vi "Unregister Event.vi"(7 "Event":refnum<class "Event.lvclass">, 8 "error in (no error)":errorcluster, 11 "View in":refnum<class "View.lvclass">) -> (0 "error out":errorcluster, 3 "View out":refnum<class "View.lvclass">)   [LabVIEW 2023, in "MVC Actors.lvlib" / "View.lvclass"]
doc: "Unregisters an event to the Controller by specifiying the concrete event."
uses:
  View.lvclass
  Event/Event.lvclass
  View.lvclass/View.ctl
  properties/Read Controller Actor Enqueuer.vi
  properties/Read Name.vi
  <vilib>/ActorFramework/Message Enqueuer/Message Enqueuer.lvclass
  Controller Messages/Unregister by Name Msg/Unregister by Name Msg.lvclass
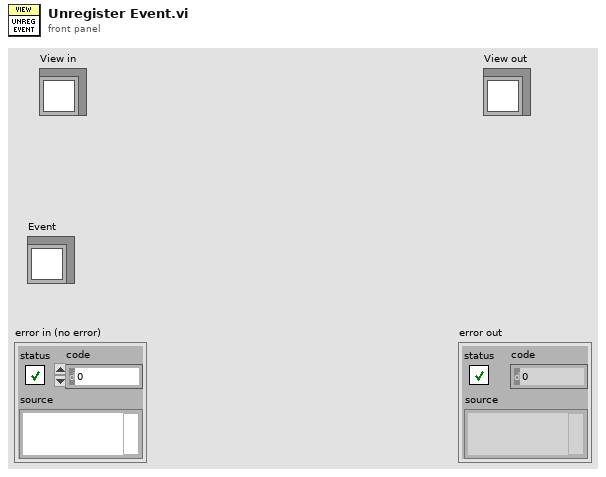
[diagram p1: front panel]
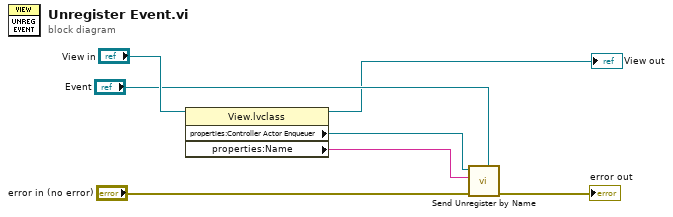
[diagram p0: block diagram]
diagram:
  n1 = property class="View.lvclass"(reference="View in") -> (reference out=→"View out":refnum<class "View.lvclass">, "properties:Controller Actor Enqueuer"=w2:refnum<class "Message Enqueuer.lvclass">, "properties:Name"=w3:string)  [unwired: 1 in, 1 out]
  n2 = call "Send Unregister by Name.vi"("Event"="Event", "error in (no error)"="error in (no error)", "View Name"=w3, "Message Enqueuer in"=w2) -> ("error out"=→"error out":errorcluster)  [unwired: 6 in, 1 out]
